vi "HardwareAcquire.vi"(8 "error in (no error)":errorcluster, 11 "ESP301.lvclass":refnum<class "ESP301.lvclass">) -> (0 "error out":errorcluster, 2 "positions":dbl[](array[numeric]), 3 "ESP301.lvclass":refnum<class "ESP301.lvclass">, 4 "motor Status":T1(array[ring]), 5 "Power Status":bool[](array[boolean]))   [LabVIEW 2020, in "ESP301.lvclass"]
uses:
  ESP301.lvclass
  stop FGV control.ctl
  AcquireTypeDef.ctl
  ESP301.lvclass/ESP301.ctl
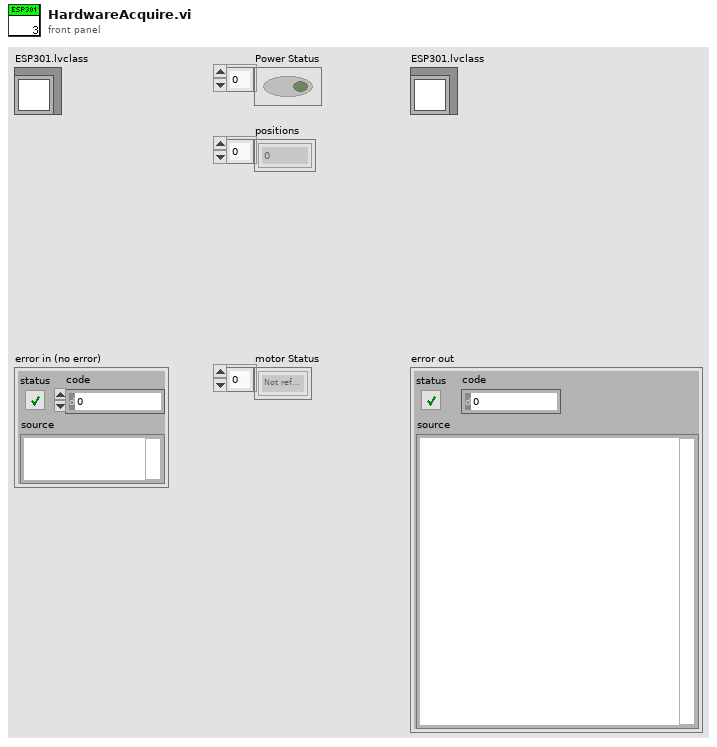
[diagram p1: front panel]
types:
  T1 = enum16{"Not referenced", "Homing", "Moving", "Ready"}[]
  T2 = typedef "AcquireTypeDef.ctl" = cluster{"busy":bool, "positions":dbl[], "Power Status":bool[], "motor Status":enum16{"Not referenced", "Homing", "Moving", "Ready"}[]}
  T3 = typedef "stop FGV control.ctl" = enum16{"Clear", "Write", "Read"}
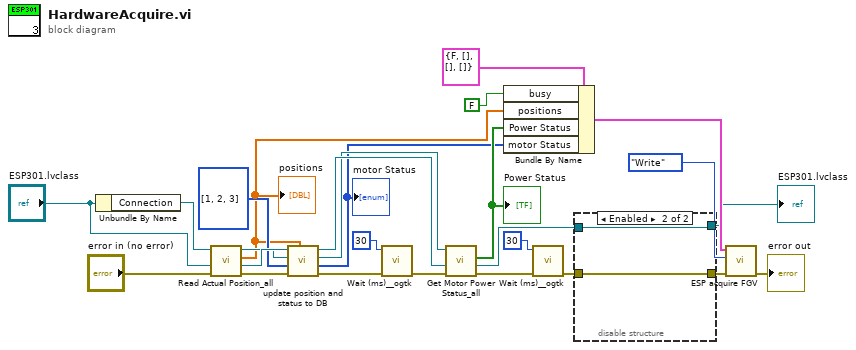
[diagram p0: block diagram]
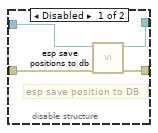
[diagram p2: hidden frame]
diagram:
  n1 = Unbundle By Name("ESP301.lvclass") -> ("Connection"=w16:refnum<visa-resource-name>)
  n2 = call-dynamic "Read Actual Position_all.vi"("error in (no error)"="error in (no error)", "ESP301"="ESP301.lvclass", "VISA resource name"=w16) -> ("error out"=w15:errorcluster, "ESP301 out"=w21:refnum<class "ESP301.lvclass">, "positions"=w11:dbl[], "VISA resource name out"=w17:refnum<visa-resource-name>)  [unwired: 1 in]
  "positions" <- w11
  n3 = call "update position and status to DB.vi"("positions"=w11, "error in (no error)"=w15, "Array in"=i32[] [1, 2, 3], "VISA resource name in"=w17, "ESP301 in"=w21) -> ("error out"=w23:errorcluster, "motor Status"=w9:T1, "VISA resource name out out"=w22:refnum<visa-resource-name>, "ESP301 out"=w26:refnum<class "ESP301.lvclass">)  [unwired: 3 in]
  "motor Status" <- w9
  n4 = call "Wait (ms)__ogtk.vi"("error in (no error)"=w23, "milliseconds to wait"=u32 30) -> ("error out"=w24:errorcluster)  [unwired: 8 in, 1 out]
  n5 = call-dynamic "Get Motor Power Status_all.vi"("error in (no error)"=w24, "ESP301 in"=w26, "VISA resource name"=w22) -> ("error out"=w2:errorcluster, "ESP301 out"=w6:refnum<class "ESP301.lvclass">, "Power Status"=w10:bool[])  [unwired: 1 in, 1 out]
  "Power Status" <- w10
  n6 = Bundle By Name(cluster=T2 {"busy"=FALSE, "positions"=[], "Power Status"=[], "motor Status"=[]} ("ESP301 Acq Data"), "busy"=FALSE, "positions"=w11, "Power Status"=w10, "motor Status"=w9) -> (w8:T2)
  n7 = call "Wait (ms)__ogtk.vi"("error in (no error)"=w2, "milliseconds to wait"=u32 30) -> ("error out"=w1:errorcluster)  [unwired: 8 in, 1 out]
  n8 = disable-structure shown="Enabled" {
    disable-tunnel: w6 -> [w30 w31]
    disable-tunnel: [w29 w31] -> w5
    disable-tunnel: [w28 w32] -> w4
    disable-tunnel: w1 -> [w27 w32]
    frame Disabled {
      # "esp save position to DB"
      n9 = call-dynamic "esp save positions to db.vi"("error in (no error)"=w27, "ESP301 in"=w30) -> ("error out"=w28:errorcluster, "ESP301 out"=w29:refnum<class "ESP301.lvclass">)  [unwired: 8 in]
    }
    frame Enabled {
    }
  }
  "ESP301.lvclass" <- w5
  n10 = call "ESP acquire FGV.vi"("error in"=w4, "Function"=stop_FGV_control."Write", "ESP301 Acq Data"=w8) -> ("error out"=→"error out":errorcluster)  [unwired: 7 in, 1 out]
